vi "PAN_ModsMgr.vi"(10 "Modules":string[](array[string])) -> (2 "response":string)   [LabVIEW 2016]
uses:
  Modules/DBSHAND/private/vis/DatabaseHand_Element_Get(bool).vi
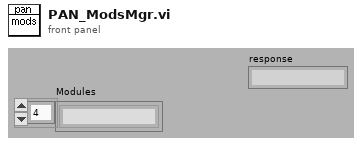
[diagram p1: front panel]
types:
  T1 = typedef "DatabaseHand_RefNum.ctl" = refnum<vi>
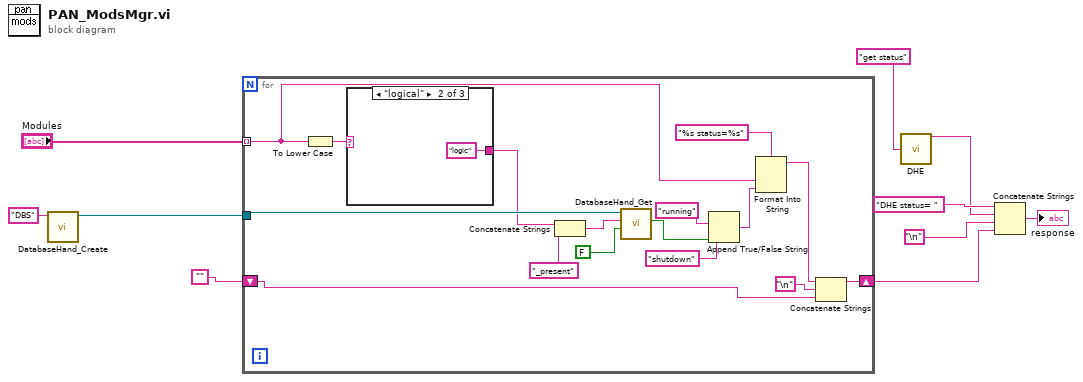
[diagram p0: block diagram]
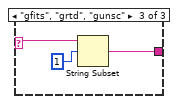
[diagram p3: hidden frame]
diagram:
  n1 = call "DatabaseHand_Create.vi"("Name"="DBS") -> ("Database RefNum out"=w8:T1)  [unwired: 1 in, 9 out]
  n2 = for {
    tunnel: "Modules" -> [w20] mode=indexing
    tunnel: w8 -> [w26]
    shift-right: [w14] -> w1
    shift-left: "" -> [w11]
    n3 = To Lower Case(string=w20) -> (all lower case string=w25:string)
    n4 = case shown="\"logical\"" w25 {
      selector: w25 -> [w27 _ w31]
      tunnel: [w27 "logic" w29] -> w24
      frame Default {
      }
      frame "logical" {
      }
      frame "gfits", "grtd", "gunsc" {
        n5 = String Subset(string=w31, offset (0)=1) -> (substring=w29:string)  [unwired: 1 out]
      }
    }
    n6 = Concatenate Strings(w24, "_present" ("string")) -> (w21:string)
    n7 = call-poly "DatabaseHand_Get.vi"("default value"=FALSE, "name"=w21, "Database RefNum in"=w26) -> ("value"=w18:bool)  [unwired: 2 in, 6 out]
    n8 = Append True/False String(1:w18, 2:"shutdown" ("false string"), 3:"running" ("true string")) -> (0:w15:string)  [unwired: 1 out]
    n9 = Format Into String(format string="%s status=%s", w20, w15) -> (resulting string=w13:string)  [unwired: 2 in, 1 out]
    n10 = Concatenate Strings(w13, "\n", w11) -> (w14:string)
  }
  n11 = call "DHE.vi"("Cmd"="get status") -> ("ImmedReplyString"=w4:string)  [unwired: 2 in, 12 out]
  n12 = Concatenate Strings("DHE status= " ("string"), w4, "\n", w1) -> (→"response":string)
